vi "G Array to PLC Byte Stream.vi"(8 "error in (no error)":errorcluster, 9 "Array Information":T1, 10 "Value":variant, 11 "TwinCAT ADS in":refnum<class "TwinCAT ADS.lvclass">) -> (0 "error out":errorcluster, 2 "Byte Stream":u8[](array[numeric]), 3 "TwinCAT ADS out":refnum<class "TwinCAT ADS.lvclass">)   [LabVIEW 2018, in "TwinCAT ADS.lvclass"]
uses:
  TwinCAT ADS.lvclass
  Controls/PLC Array Type Descriptor.ctl
  Controls/PLC Type.ctl
  Controls/PLC Sub-Item Type Descriptor.ctl
  G Primitive to PLC Byte Stream.vi/ebfc1059-5ad7-41af-9a32-6ba056cec1e2.vi
  G Primitive to PLC Byte Stream.vi/6e01a951-886b-41b5-8cd1-fdd71fd1a533.vi
  G Primitive to PLC Byte Stream.vi/09c7a0ef-3209-4624-b801-f77696e71225.vi
  G Primitive to PLC Byte Stream.vi/97b8602c-6a72-408e-90bf-08a26de32539.vi
  G Primitive to PLC Byte Stream.vi/0fd4fbf3-4a18-432c-8f70-6a5c8fef8454.vi
  G Primitive to PLC Byte Stream.vi/afdb5a5e-237c-4be5-828e-15f510cf6cea.vi
  G Primitive to PLC Byte Stream.vi/185a6e12-4d7d-4ad7-9936-0525adb2f85e.vi
  G Primitive to PLC Byte Stream.vi/88229fb8-b58c-494b-bd2b-fea6e0d0ed1b.vi
  G Primitive to PLC Byte Stream.vi/e57df404-389c-41d0-a67c-37c75754ab31.vi
  G Primitive to PLC Byte Stream.vi/d0ee652c-9b86-46ed-9065-57d03aa8de3e.vi
  G Primitive to PLC Byte Stream.vi/886bf0b9-f01c-4a44-b2e2-abccc7b97bfa.vi
  G Primitive to PLC Byte Stream.vi/35f71df7-fc14-4c4d-983c-cf72c138dc9e.vi
  G Primitive to PLC Byte Stream.vi/2d2bc992-a9ff-4dd8-b8fe-74c21cb85899.vi
  G Primitive to PLC Byte Stream.vi/100e4a11-5e4a-45b7-be98-adc9eaebd48d.vi
  G Primitive to PLC Byte Stream.vi/132946d9-68c7-4ade-a66d-dc369520c644.vi
  <vilib>/Utility/error.llb/Trim Whitespace.vi
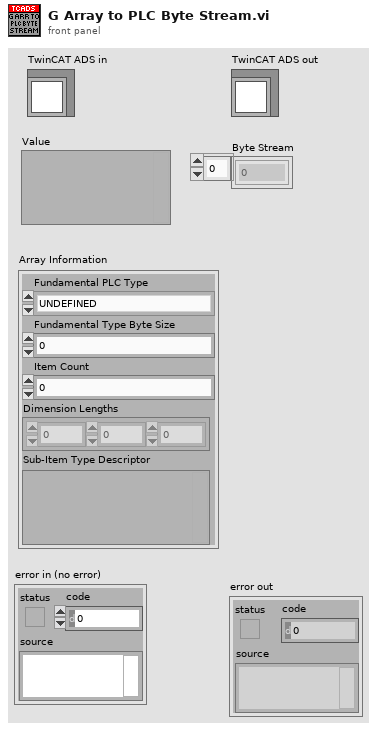
[diagram p1: front panel]
types:
  T1 = typedef "TwinCAT ADS.lvclass/PLC Array Type Descriptor.ctl" = cluster{"Fundamental PLC Type":T2, "Fundamental Type Byte Size":i32, "Item Count":i32, "Dimension Lengths":i32[], "Sub-Item Type Descriptor":variant}
  T2 = typedef "TwinCAT ADS.lvclass/PLC Type.ctl" = enum16{"UNDEFINED", "INT", "DINT", "REAL", "LREAL", "SINT", "BYTE", "UINT", "UDINT", "LINT", "ULINT", "STRING", "WSTRING", "BOOL", "TIME", "LTIME", "DATE", "DT", "TOD", "ARRAY", "JAGGED ARRAY", "STRUCT", "FUNCTION BLOCK", "UNION", "POINTER", "USER DEFINED"}
  T3 = typedef "TwinCAT ADS.lvclass/PLC Sub-Item Type Descriptor.ctl" = cluster{"PLC Type":T2, "Offset":i32, "Byte Size":i32, "[Sub-Item/Array Type Descriptor]":variant[]}
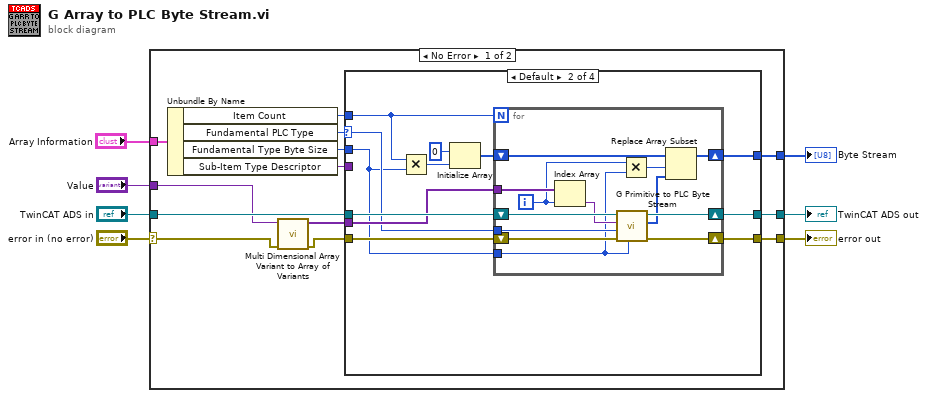
[diagram p0: block diagram]
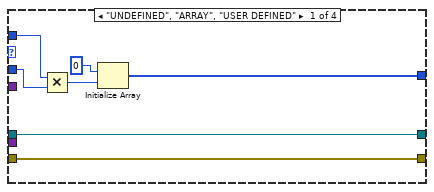
[diagram p2: hidden frame]
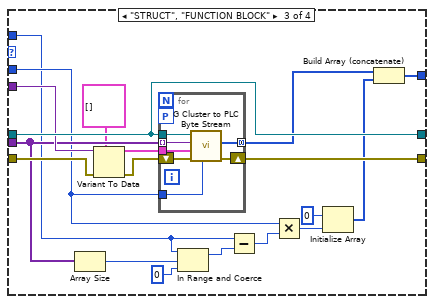
[diagram p3: hidden frame]
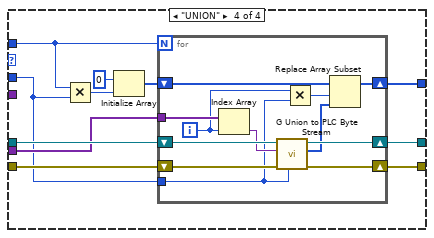
[diagram p4: hidden frame]
diagram:
  n1 = case shown="No Error" "error in (no error)" {
    selector: "error in (no error)" -> [w9 w103]
    tunnel: "TwinCAT ADS in" -> [w20 w102]
    tunnel: [w19 w102] -> w6
    tunnel: "Array Information" -> [w18 _]
    tunnel: [w16 _] -> w4
    tunnel: [w11 w103] -> w3
    tunnel: "Value" -> [w10 _]
    frame No Error {
      n2 = Unbundle By Name(w18) -> ("Item Count"=w8:i32, "Fundamental PLC Type"=w13:T2, "Fundamental Type Byte Size"=w12:i32, "Sub-Item Type Descriptor"=w17:variant)
      n3 = call "Multi Dimensional Array Variant to Array of Variants.vi"("error in (no error)"=w9, "Array Variant"=w10) -> ("error out"=w15:errorcluster, "[Variant]"=w14:variant[])  [unwired: 8 in]
      n4 = case shown="Default" w13 {
        selector: w13 -> [_ w33 _ _]
        tunnel: w15 -> [w27 w37 w70 w87]
        tunnel: w20 -> [w26 w39 w71 w89]
        tunnel: [w27 w36 w68 w86] -> w11
        tunnel: [w26 w35 w71 w85] -> w19
        tunnel: w17 -> [_ _ w69 _]
        tunnel: [w23 w34 w60 w84] -> w16
        tunnel: w14 -> [_ w38 w67 w88]
        tunnel: w12 -> [w21 w32 w57 w83]
        tunnel: w8 -> [w22 w31 w53 w82]
        frame "UNDEFINED", "ARRAY", "USER DEFINED" {
          n5 = Multiply(x=w22, y=w21) -> (x*y=w24:i32)
          n6 = Initialize Array(u8 0, w24) -> (w23:u8[])
        }
        frame Default {
          n7 = Multiply(x=w31, y=w32) -> (x*y=w30:i32)
          n8 = Initialize Array(u8 0, w30) -> (w28:u8[])
          n9 = for {
            N: w31 -> [_]
            shift-right: [w49] -> w35
            shift-left: w39 -> [w52]
            shift-right: [w50] -> w36
            shift-left: w37 -> [w51]
            tunnel: w38 -> [w47]
            shift-right: [w44] -> w34
            shift-left: w28 -> [w45]
            tunnel: w32 -> [w42]
            tunnel: w33 -> [w48]
            i -> [w41]
            n10 = Index Array(array=w47, index=w41) -> (element=w46:variant)
            n11 = call "G Primitive to PLC Byte Stream.vi"("Byte Length"=w42, "error in (no error)"=w51, "PLC Type"=w48, "Value"=w46, "TwinCAT ADS in"=w52) -> ("error out"=w50:errorcluster, "Byte Stream"=w43:u8[], "TwinCAT ADS out"=w49:refnum<class "TwinCAT ADS.lvclass">)  [unwired: 4 in]
            n12 = Multiply(x=w41, y=w42) -> (x*y=w40:i32)
            n13 = Replace Array Subset(array=w45, new element=w43, index=w40) -> (w44:u8[])
          }
        }
        frame "STRUCT", "FUNCTION BLOCK" {
          n14 = Array Size(array=w67) -> (size(s)=w55:i32)
          n15 = Variant To Data(error in=w70, type=T3[] [] ("[Sub-Item Type Information]"), Variant=w69) -> (data=w64:T3[], error out=w66:errorcluster)
          n16 = for {
            tunnel: w64 -> [w76]
            tunnel: w67 -> [w72] mode=indexing
            shift-right: [w74] -> w68
            shift-left: w66 -> [w78]
            tunnel: w57 -> [w75]
            tunnel: [w73] -> w62 mode=concatenating
            workers-P: _ -> [_]
            tunnel: w71 -> [w77]
            n17 = call "G Cluster to PLC Byte Stream.vi"("Byte Length"=w75, "error in (no error)"=w78, "[Sub-Item Type Descriptor]"=w76, "Value"=w72, "TwinCAT ADS in"=w77) -> ("error out"=w74:errorcluster, "Byte Stream"=w73:u8[])  [unwired: 4 in, 1 out]
          }
          n18 = In Range and Coerce(upper limit=w53, x=w55, lower limit=0) -> (coerced(x)=w56:i32)  [unwired: 1 out]
          n19 = Subtract(x=w53, y=w56) -> (x-y=w59:i32)
          n20 = Multiply(x=w57, y=w59) -> (x*y=w58:i32)
          n21 = Initialize Array(u8 0, w58) -> (w63:u8[])
          n22 = Build Array (concatenate)(w62, w63) -> (w60:u8[])
        }
        frame "UNION" {
          n23 = Multiply(x=w82, y=w83) -> (x*y=w81:i32)
          n24 = Initialize Array(u8 0, w81) -> (w79:u8[])
          n25 = for {
            N: w82 -> [_]
            shift-right: [w99] -> w85
            shift-left: w89 -> [w100]
            shift-right: [w93] -> w86
            shift-left: w87 -> [w101]
            tunnel: w88 -> [w98]
            shift-right: [w96] -> w84
            shift-left: w79 -> [w97]
            tunnel: w83 -> [w90]
            i -> [w95]
            n26 = Index Array(array=w98, index=w95) -> (element=w92:variant)
            n27 = call "G Union to PLC Byte Stream.vi"("Byte Length"=w90, "error in (no error)"=w101, "Value"=w92, "TwinCAT ADS in"=w100) -> ("error out"=w93:errorcluster, "Byte Stream"=w91:u8[], "TwinCAT ADS out"=w99:refnum<class "TwinCAT ADS.lvclass">)  [unwired: 5 in]
            n28 = Multiply(x=w95, y=w90) -> (x*y=w94:i32)
            n29 = Replace Array Subset(array=w97, new element=w91, index=w94) -> (w96:u8[])
          }
        }
      }
    }
    frame Error {
    }
  }
  "error out" <- w3
  "Byte Stream" <- w4
  "TwinCAT ADS out" <- w6
